vi "DistanceFromTarget.vi"(8 "ty Limelight":dbl, 9 "Altura da lente":dbl, 10 "Ângulo de montagem":dbl, 11 "Altura do alvo":dbl) -> (3 "Distance From the Target":dbl)   [LabVIEW 2020]
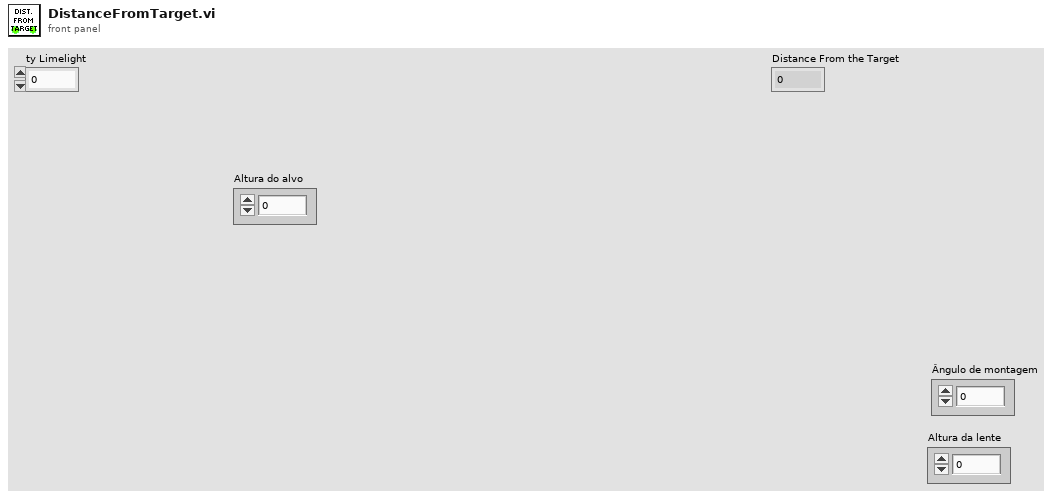
[diagram p1: front panel]
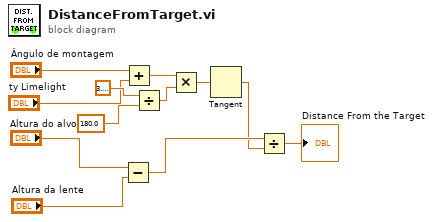
[diagram p0: block diagram]
diagram:
  n1 = Subtract(x="Altura do alvo", y="Altura da lente") -> (x-y=w5:dbl)
  n2 = Add(x="Ângulo de montagem", y="ty Limelight") -> (x+y=w11:dbl)
  n3 = Divide(x=3.141592653589793, y=180.0) -> (x/y=w8:dbl)
  n4 = Multiply(x=w11, y=w8) -> (x*y=w4:dbl)
  n5 = Tangent(1:w4) -> (0:w3:dbl)
  n6 = Divide(x=w5, y=w3) -> (x/y=→"Distance From the Target":dbl)
